vi "Verify File Exists and Not Empty.vi"(8 "error in":errorcluster, 11 "path":path) -> (0 "error out":errorcluster)   [LabVIEW 2024]
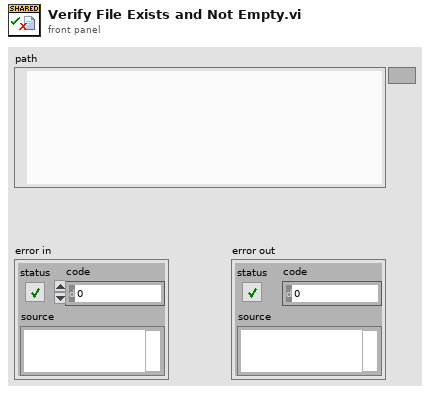
[diagram p1: front panel]
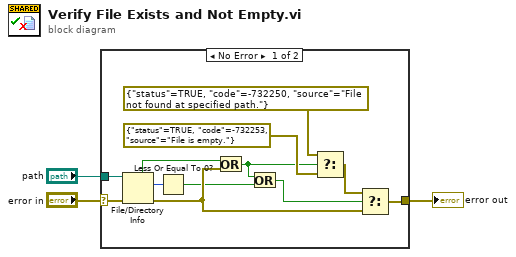
[diagram p0: block diagram]
diagram:
  n1 = case shown="No Error" "error in" {
    selector: "error in" -> [w12 w16]
    tunnel: [w15 w16] -> w1
    tunnel: "path" -> [w13 _]
    frame No Error {
      n2 = File/Directory Info(path=w13, error in=w12) -> (directory=w8:bool, size=w14:i64, error out=w7:errorcluster)  [unwired: 4 out]
      n3 = Less Or Equal To 0?(x=w14) -> (x <= 0?=w5:bool)
      n4 = Or(x=w8, y=w7) -> (x .or. y?=w6:bool)
      n5 = Or(x=w6, y=w5) -> (x .or. y?=w4:bool)
      n6 = Select(t=errorcluster {"status"=TRUE, "code"=-732250, "source"="File not found at specified path."} ("f"), s=w6, f=errorcluster {"status"=TRUE, "code"=-732253, "source"="File is empty."}) -> (s? t:f=w9:errorcluster)
      n7 = Select(t=w9, s=w4, f=w7) -> (s? t:f=w15:errorcluster)
    }
    frame Error {
    }
  }
  "error out" <- w1
